vi "getTelemetryHardpointStatus.vi"(11 "Publisher in":refnum<class "Publisher.lvclass">) -> (2 "TelemetryHardpointStatus":T1, 3 "Publisher out":refnum<class "Publisher.lvclass">)   [LabVIEW 2016, in "Publisher.lvclass"]
uses:
  Publisher.lvclass
  DataTypes/Topics/TelemetryHardpointStatus.ctl
  DataTypes/Topics/Parts/Timestamp.ctl
  Publisher.lvclass/Publisher.ctl
  DataTypes/Topics/M1M3SupportTopics.lvlib
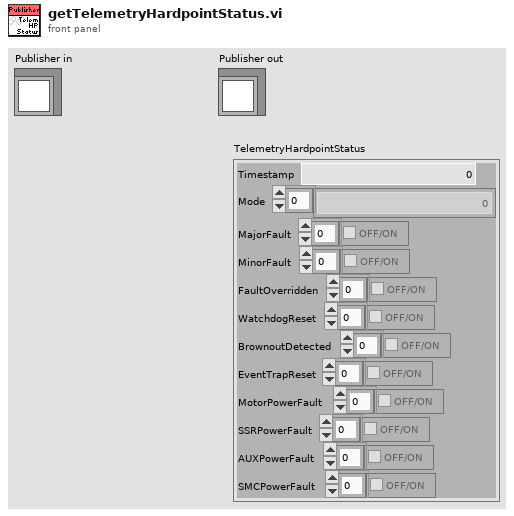
[diagram p1: front panel]
types:
  T1 = typedef "M1M3SupportTopics.lvlib/TelemetryHardpointStatus.ctl" = cluster{"Timestamp":T2, "Mode":u8[], "MajorFault":bool[], "MinorFault":bool[], "FaultOverridden":bool[], "WatchdogReset":bool[], "BrownoutDetected":bool[], "EventTrapReset":bool[], "MotorPowerFault":bool[], "SSRPowerFault":bool[], "AUXPowerFault":bool[], "SMCPowerFault":bool[]}
  T2 = typedef "M1M3SupportTopics.lvlib/Timestamp.ctl" = dbl
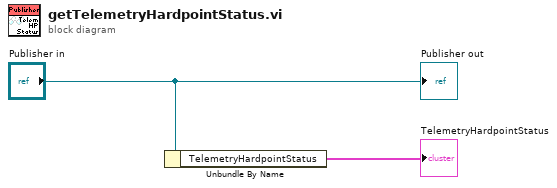
[diagram p0: block diagram]
diagram:
  n1 = Unbundle By Name("Publisher in") -> ("TelemetryHardpointStatus"=→"TelemetryHardpointStatus":T1)
  "Publisher out" <- "Publisher in"
